vi "All Functions.vi"() -> ()   [LabVIEW 2012]
uses:
  Controls/Bulk Wrapper Action.ctl
panel:
  in  "Boolean":bool
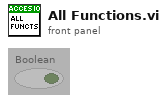
[diagram p1: front panel]
types:
  T1 = typedef "Bulk Wrapper Action.ctl" = enum16{"Start Read", "Read Buffer"}
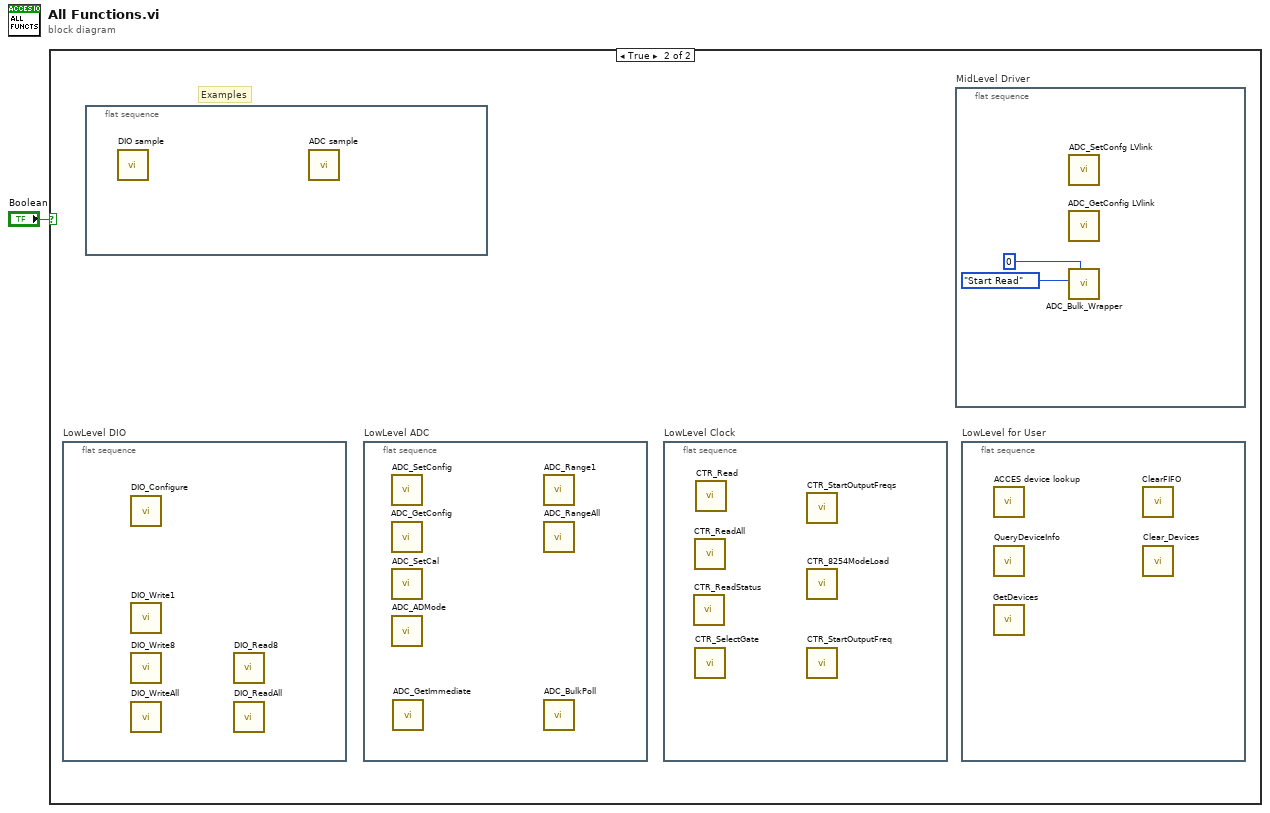
[diagram p0: block diagram]
diagram:
  n1 = case shown="True" "Boolean" {
    frame False {
    }
    frame True {
      # "Examples"
      n2 = flat-sequence "LowLevel DIO" {
        frame #0 {
          n3 = call "DIO_Configure.vi"() -> ()  [unwired: 11 in, 1 out]
          n4 = call "DIO_Write1.vi"() -> ()  [unwired: 11 in, 1 out]
          n5 = call "DIO_Write8.vi"() -> ()  [unwired: 11 in, 1 out]
          n6 = call "DIO_WriteAll.vi"() -> ()  [unwired: 11 in, 1 out]
          n7 = call "DIO_Read8.vi"() -> ()  [unwired: 12 in]
          n8 = call "DIO_ReadAll.vi"() -> ()  [unwired: 9 in, 3 out]
        }
      }
      n9 = flat-sequence {
        frame #0 {
          n10 = call "DIO sample.vi"() -> ()  [unwired: 1 in]
          n11 = call "ADC sample.vi"() -> ()  [unwired: 15 in, 1 out]
        }
      }
      n12 = flat-sequence "LowLevel ADC" {
        frame #0 {
          n13 = call "ADC_SetConfig.vi"() -> ()  [unwired: 10 in, 2 out]
          n14 = call "ADC_GetConfig.vi"() -> ()  [unwired: 9 in, 3 out]
          n15 = call "ADC_SetCal.vi"() -> ()  [unwired: 11 in, 1 out]
          n16 = call "ADC_ADMode.vi"() -> ()  [unwired: 11 in, 1 out]
          n17 = call "ADC_GetImmediate.vi"() -> ()  [unwired: 10 in, 2 out]
          n18 = call "ADC_Range1.vi"() -> ()  [unwired: 11 in, 1 out]
          n19 = call "ADC_RangeAll.vi"() -> ()  [unwired: 11 in, 1 out]
          n20 = call "ADC_BulkPoll.vi"() -> ()  [unwired: 10 in, 2 out]
        }
      }
      n21 = flat-sequence "LowLevel Clock" {
        frame #0 {
          n22 = call "CTR_ReadStatus.vi"() -> ()  [unwired: 11 in, 1 out]
          n23 = call "CTR_ReadAll.vi"() -> ()  [unwired: 11 in, 1 out]
          n24 = call "CTR_SelectGate.vi"() -> ()  [unwired: 11 in, 1 out]
          n25 = call "CTR_Read.vi"() -> ()  [unwired: 11 in, 1 out]
          n26 = call "CTR_StartOutputFreqs.vi"() -> ()  [unwired: 9 in, 3 out]
          n27 = call "CTR_8254ModeLoad.vi"() -> ()  [unwired: 9 in, 3 out]
          n28 = call "CTR_StartOutputFreq.vi"() -> ()  [unwired: 10 in, 2 out]
        }
      }
      n29 = flat-sequence "MidLevel Driver" {
        frame #0 {
          n30 = call "ADC_SetConfg LVlink.vi"() -> ()  [unwired: 11 in, 1 out]
          n31 = call "ADC_GetConfig LVlink.vi"() -> ()  [unwired: 5 in, 7 out]
          n32 = call "ADC_Bulk_Wrapper.vi"("DeviceIndex"=u32 0, "Action"=Bulk_Wrapper_Action."Start Read" ("Enum")) -> ()  [unwired: 6 in, 4 out]
        }
      }
      n33 = flat-sequence "LowLevel for User" {
        frame #0 {
          n34 = call "ACCES device lookup.vi"() -> ()  [unwired: 10 in, 2 out]
          n35 = call "QueryDeviceInfo.vi"() -> ()  [unwired: 1 in, 4 out]
          n36 = call "GetDevices.vi"() -> ()  [unwired: 1 out]
          n37 = call "ClearFIFO.vi"() -> ()  [unwired: 11 in, 1 out]
          n38 = call "Clear_Devices.vi"() -> ()  [unwired: 11 in, 1 out]
        }
      }
    }
  }
